vi "Close Application Reference.vi"(8 "error in (no error)":errorcluster, 11 "App Control API in":refnum<class "AppControlAPI.lvclass">) -> (0 "error out":errorcluster, 3 "App Control API out":refnum<class "AppControlAPI.lvclass">)   [LabVIEW 2018, in "AppControlAPI.lvclass"]
uses:
  AppControlAPI.lvclass
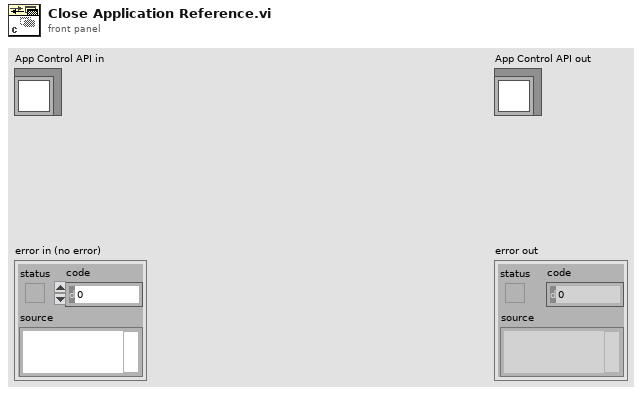
[diagram p1: front panel]
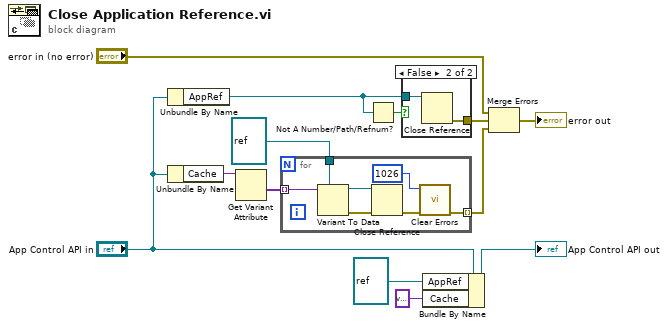
[diagram p0: block diagram]
diagram:
  n1 = Unbundle By Name("App Control API in") -> ("AppRef"=w1:refnum<vi>)
  n2 = Unbundle By Name("App Control API in") -> ("Cache"=w2:variant)
  n3 = Get Variant Attribute(Variant=w2) -> (values=w4:variant[])  [unwired: 3 in, 3 out]
  n4 = for {
    tunnel: w4 -> [w17] mode=indexing
    tunnel: refnum<vi> refnum ("This VI") -> [w20]
    tunnel: [w16] -> w5 mode=indexing
    n5 = Variant To Data(type=w20, Variant=w17) -> (data=w19:refnum<vi>, error out=w14:errorcluster)  [unwired: 1 in]
    n6 = Close Reference(reference=w19, error in (no error)=w14) -> (error out=w18:errorcluster)
    n7 = call <vilib>:"Clear Errors.vi"("error in (no error)"=w18, "specific error code to clear (0: all)"=1026) -> ("error out"=w16:errorcluster)  [unwired: 4 in, 1 out]
  }
  n8 = Not A Number/Path/Refnum?(number/path/refnum=w1) -> (NaN/Path/Refnum?=w12:bool)
  n9 = case shown="False" w12 {
    tunnel: w1 -> [_ w21]
    tunnel: [_ w22] -> w9
    frame True {
    }
    frame False {
      n10 = Close Reference(reference=w21) -> (error out=w22:errorcluster)  [unwired: 1 in]
    }
  }
  n11 = Bundle By Name(cluster="App Control API in", "AppRef"=refnum<vi> refnum, "Cache"=variant ("Variant")) -> (→"App Control API out":refnum<class "AppControlAPI.lvclass">)
  n12 = Merge Errors("error in (no error)", w9, w5) -> (→"error out":errorcluster)
